vi "全局初始化.vi"   [LabVIEW 2014]
types:
  T1 = cluster{"有功常数":i32, "无功常数":i32, "校验圈数":i32, "校验类型":i32, "S值计算次数":i32, "S值计算方法":i32}
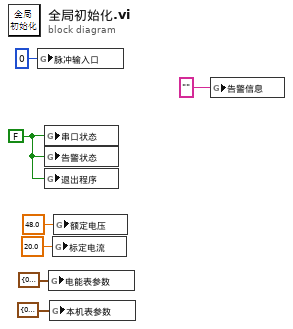
[diagram p0: block diagram]
diagram:
  w6 = FALSE ("串口锁")
  n1 = global write "程序全局.vi" "脉冲输入口"(u8 0 ("脉冲输入口")) -> ()
  n2 = global write "系统全局.vi" "串口状态"(w6) -> ()
  n3 = global write "系统全局.vi" "告警状态"(w6) -> ()
  n4 = global write "系统全局.vi" "退出程序"(w6) -> ()
  n5 = global write "程序全局.vi" "电能表参数"(T1 {"有功常数"=0, "无功常数"=0, "校验圈数"=0, "校验类型"=0, "S值计算次数"=0, "S值计算方法"=0} ("电能表参数")) -> ()
  n6 = global write "程序全局.vi" "本机表参数"(cluster{"有功常数":i32, "无功常数":i32, "输出类型":i32} {"有功常数"=0, "无功常数"=0, "输出类型"=0} ("本机表参数")) -> ()
  n7 = global write "程序全局.vi" "标定电流"(sgl 20.0 ("标定电流")) -> ()
  n8 = global write "程序全局.vi" "额定电压"(sgl 48.0 ("额定电压")) -> ()
  n9 = global write "系统全局.vi" "告警信息"("" ("发送缓冲")) -> ()
